vi "uSubscriber Register.vi"(8 "error in (no error)":errorcluster, 9 "Policy (All-Topics)":refnum<class "uPolicy.lvclass">, 10 "Broker":refnum<class "uTransport_uActor.lvclass">, 11 "Subscriber's uTransport":refnum<class "uTransport.lvclass">) -> (0 "error out":errorcluster)   [LabVIEW 2021, in "uFramework.lvlib" / "uClient_Subscriber.lvclass"]
uses:
  uClient_Subscriber.lvclass
  uTransport_uActor/uTransport_uActor.lvclass
  U:/Projects/uFramework/Src/uFramework/uTransport/uTransport.lvclass
  uTransport/uTransport.lvclass
  uPolicy/uPolicy.lvclass
  Bin/uData.lvlibp/uData.lvclass
  uMsg/uMsg.lvclass
  U:/Projects/uFramework/Src/uFramework/uClient/uClient.lvclass
  uClient_Subscriber.lvclass/uClient_Subscriber.ctl
  uTransport_Queue/uTransport_Queue.lvclass/uTransport_Queue.ctl
  uMsg/uMsg.lvclass/uMsg.ctl
  uClient/uClient.lvclass/uClient.ctl
  uMsg/uMsg Get Payload.vi
  uTransport/uTransport_SendMsg.vi
  uTransport_Queue/uTransport_Queue_Create.vi
  uMsg/uMsg Update Timestamp.vi
  uTransport_Queue/uTransport_Queue.lvclass
  <vilib>/Utility/error.llb/Error Cluster From Error Code.vi
  uClient/uClient.lvclass
  uNotifyMode/uNotifyMode.lvclass
  U:/Projects/uFramework/Src/uFramework/uClient_Subscriber/uClient_Subscriber.lvclass
  U:/Projects/uFramework/Src/uFramework/uTransport_uActor/uTransport_uActor.lvclass
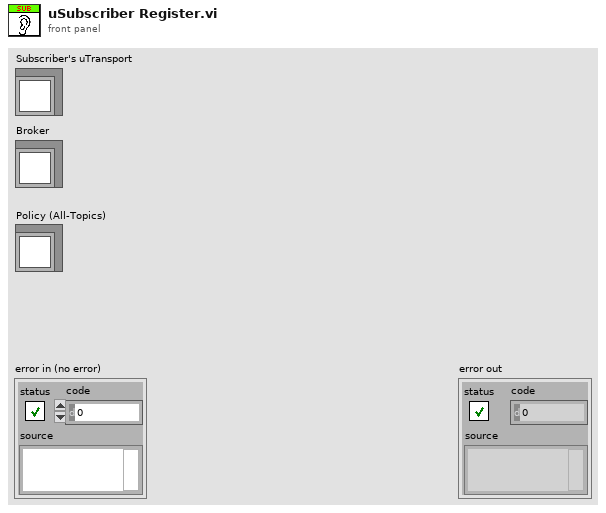
[diagram p1: front panel]
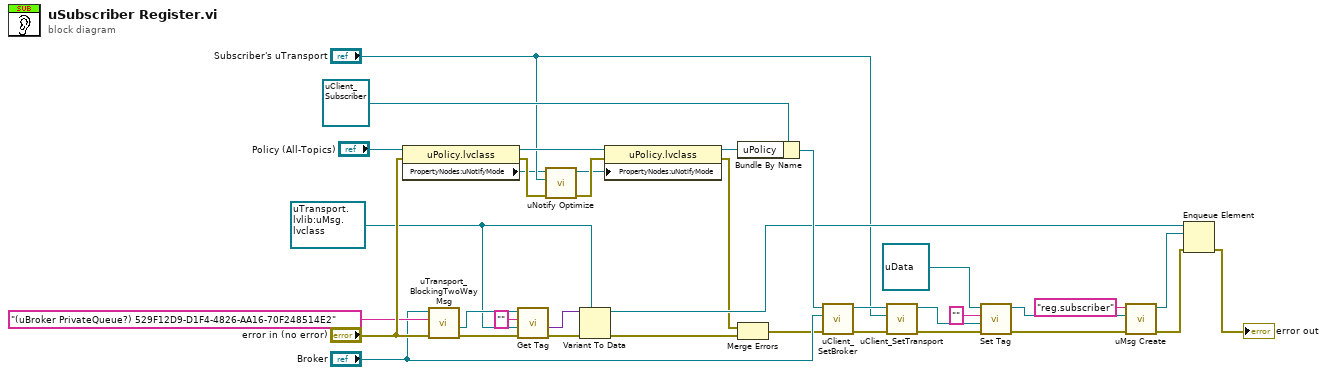
[diagram p0: block diagram]
diagram:
  w23 = refnum<queue> refnum ("brokerage queue")
  n1 = property class="uPolicy.lvclass"(reference="Policy (All-Topics)", error in="error in (no error)") -> (reference out=w8:refnum<class "uPolicy.lvclass">, error out=w33:errorcluster, "PropertyNodes:uNotifyMode"=w1:refnum<class "uNotifyMode.lvclass">)
  n2 = call "uTransport_BlockingTwoWayMsg.vi"("error in (no error)"="error in (no error)", "Command"="(uBroker PrivateQueue?) 529F12D9-D1F4-4826-AA16-70F248514E2", "uTransport in"="Broker") -> ("error out"=w27:errorcluster, "Reply"=w28:refnum<class "uData.lvclass">)  [unwired: 7 in]
  n3 = call "Get Tag.vi"("error in (no error)"=w27, "default value"=w23, "tag (case insensitive)"="", "uData in"=w28) -> ("error out"=w26:errorcluster, "value"=w24:variant)  [unwired: 4 in, 2 out]
  n4 = call "uNotify Optimize.vi"("error in (no error)"=w33, "Listener Transport"="Subscriber's uTransport", "uNotifyMode in"=w1) -> ("error out"=w34:errorcluster, "uNotifyMode out"=w6:refnum<class "uNotifyMode.lvclass">)  [unwired: 7 in]
  n5 = Variant To Data(error in=w26, type=w23, Variant=w24) -> (data=w20:refnum<queue>, error out=w5:errorcluster)
  n6 = property class="uPolicy.lvclass"(reference=w8, error in=w34, "PropertyNodes:uNotifyMode"=w6) -> (reference out=w7:refnum<class "uPolicy.lvclass">, error out=w3:errorcluster)
  n7 = Bundle By Name(cluster=refnum<class "uClient_Subscriber.lvclass"> refnum ("uClient_Subscriber in"), "uPolicy"=w7) -> (w29:refnum<class "uClient_Subscriber.lvclass">)
  n8 = Merge Errors(w3, w5) -> (w4:errorcluster)
  n9 = call "uClient_SetBroker.vi"("error in (no error)"=w4, "Broker"="Broker", "uClient in"=w29) -> ("error out"=w31:errorcluster, "uClient out"=w32:refnum<class "uClient_Subscriber.lvclass">)  [unwired: 7 in]
  n10 = call "uClient_SetTransport.vi"("error in (no error)"=w31, "uTransport"="Subscriber's uTransport", "uClient in"=w32) -> ("error out"=w15:errorcluster, "uClient out"=w10:refnum<class "uClient_Subscriber.lvclass">)  [unwired: 7 in]
  n11 = call "Set Tag.vi"("error in (no error)"=w15, "Variant"=w10, "tag (case insensitive)"="", "uData in"=refnum<class "uData.lvclass"> refnum) -> ("error out"=w14:errorcluster, "uData out"=w13:refnum<class "uData.lvclass">)  [unwired: 5 in, 1 out]
  n12 = call "uMsg Create.vi"("error in (no error)"=w14, "Payload"=w13, "CMD"="reg.subscriber") -> ("error out"=w17:errorcluster, "uMsg out"=w18:refnum<class "uMsg.lvclass">)  [unwired: 7 in]
  n13 = Enqueue Element(queue=w20, element=w18, error in (no error)=w17) -> (error out=→"error out":errorcluster)  [unwired: 1 in, 2 out]
